vi "Waveform generation.vi"(0 "Number of Steps":dbl, 1 "488 LASER Intensity":dbl, 2 "SPIMA Obj Ampl":dbl, 3 "SPIMB Z- galvo amplitude":dbl, 4 "SPIMA Z-Galvo Offset":dbl, 5 "SPIMA Z-Galvo Amplitude":dbl, 6 "SPIMA Camera trigger":dbl, 7 "SPIMA Objective Offset":dbl, 8 "SPIMB Objective Offset":dbl, 9 "SPIMA Y-Galvo Offset":dbl, 10 "SPIMB Camera Trigger":dbl, 11 "561 Laser Amplitude":dbl, 14 "SPIMB Objective Amplitude":dbl, 15 "SPIMA Y-Galvo Amplitude":dbl, 21 "SPIMB Z-offset":dbl, 24 "SPIMB Y Offset":dbl, 25 "SPIMB Y Amplitude":dbl) -> (20 "DAQ 2":waveform(dbl)[](array[waveform]), 27 "DAQ1":waveform(dbl)[](array[waveform]))   [LabVIEW 2016]
uses:
  <vilib>/Waveform/WDTOps.llb/WDT Append Waveforms DBL.vi
  <vilib>/measure/NI_MABase.lvlib
panel:
  # "Phase 1"
  # "Phase 2"
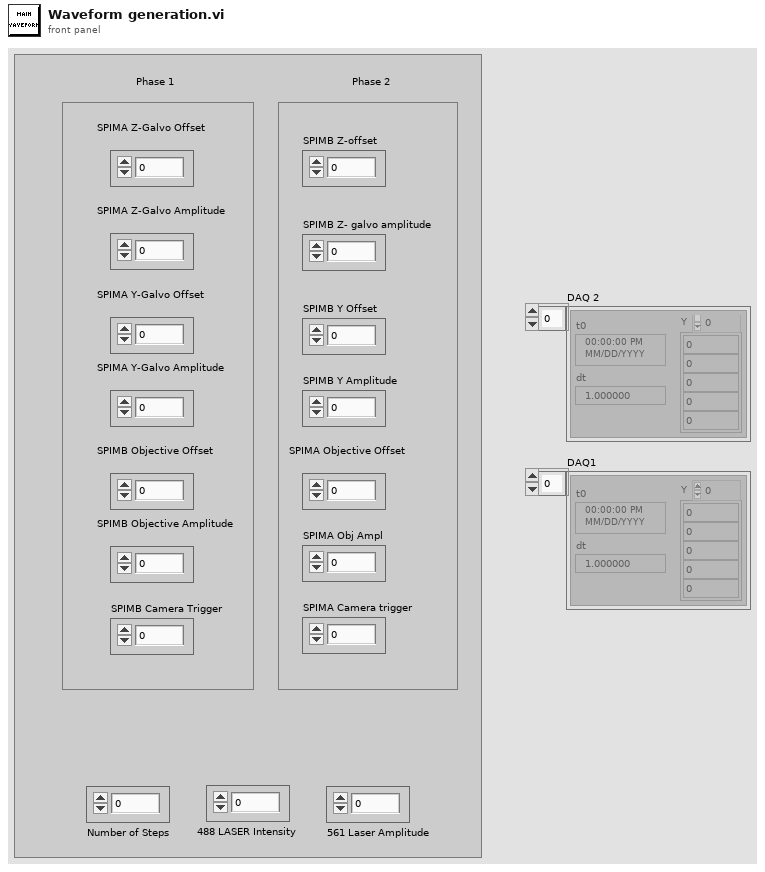
[diagram p1: front panel]
types:
  T1 = enum16{"Sine Wave", "Triangle Wave", "Square Wave", "Sawtooth Wave"}
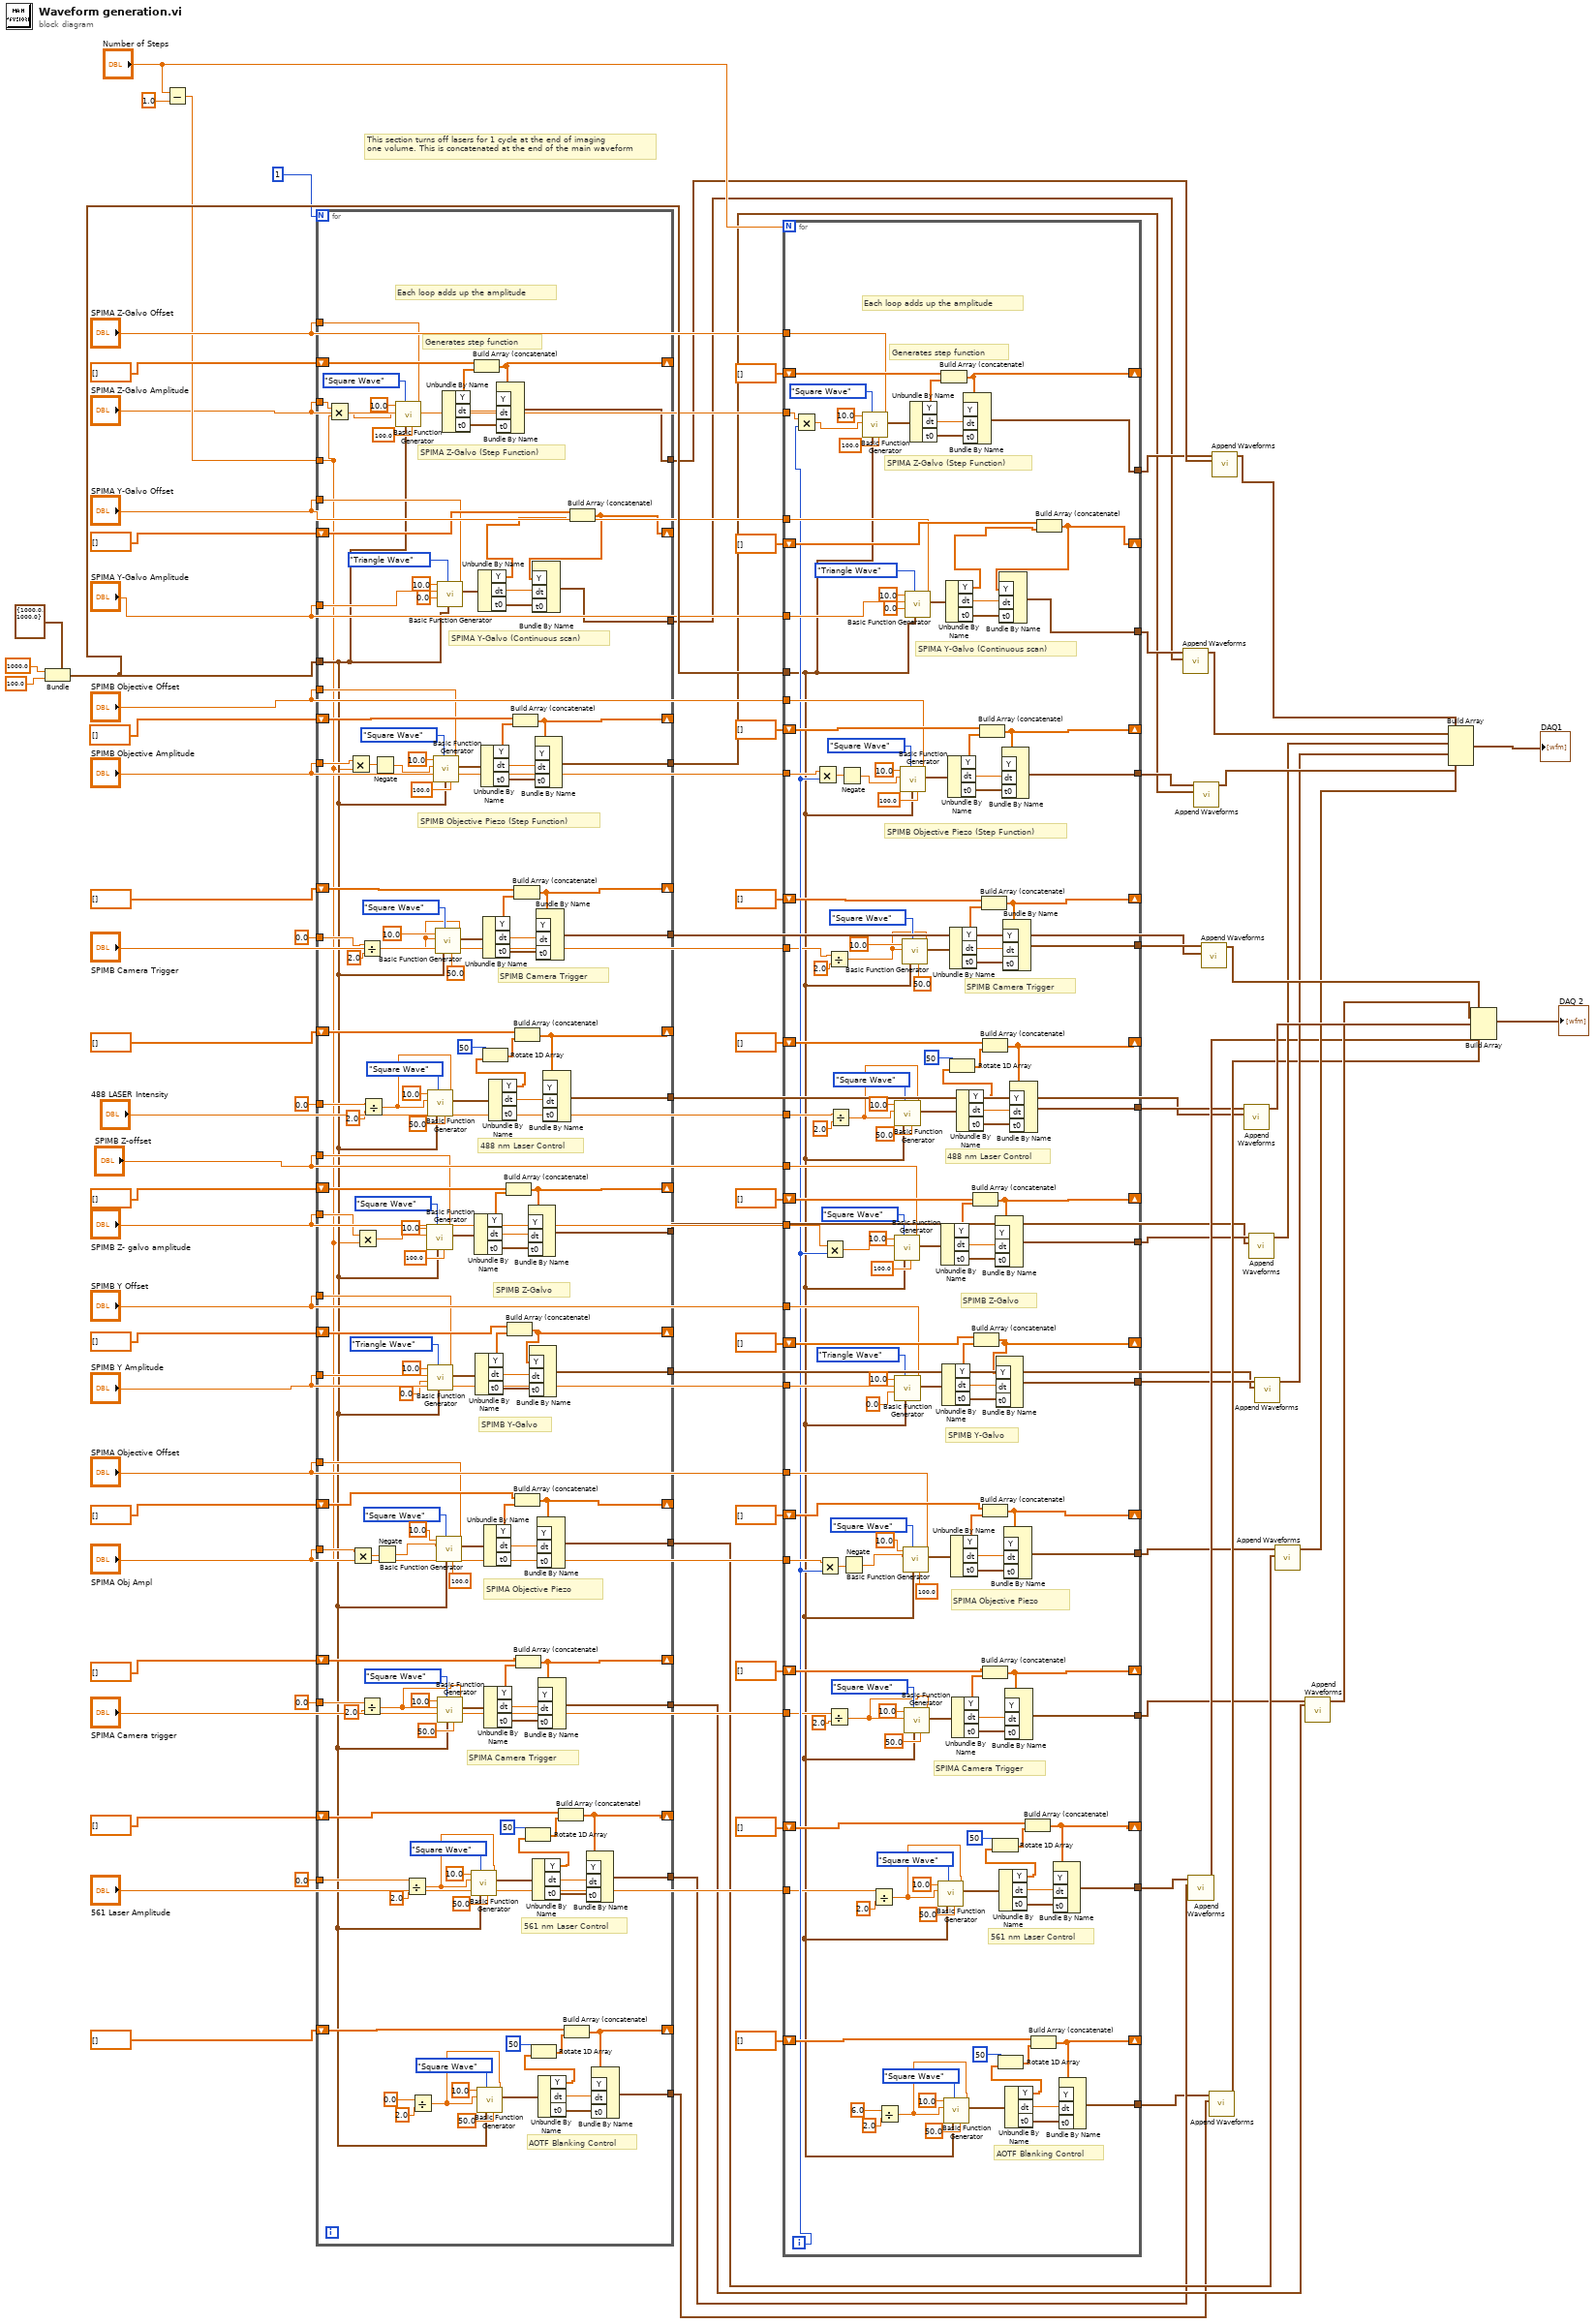
[diagram p0: block diagram]
diagram:
  # "This section turns off lasers for 1 cycle at the end of imaging\none volume. This is concatenated at the end of the main waveform"
  n1 = Bundle(cluster=cluster{"Fs":dbl, "#s":dbl} {"Fs"=1000.0, "#s"=1000.0} ("sampling info"), "Fs"=1000.0, "#s"=100.0) -> (w72:cluster{"Fs":dbl, "#s":dbl})
  n2 = Subtract(x="Number of Steps", y=1.0) -> (x-y=w29:dbl)
  n3 = for {
    N: 1 -> [_]
    shift-right: [w228] -> _
    shift-left: dbl[] [] ("appended array") -> [w229]
    tunnel: [w227] -> w22
    shift-right: [w222] -> _
    shift-left: dbl[] [] ("appended array") -> [w223]
    tunnel: [w221] -> w19
    tunnel: w72 -> [w93]
    shift-right: [w196] -> _
    shift-left: dbl[] [] ("appended array") -> [w197]
    tunnel: [w195] -> w17
    shift-right: [w193] -> _
    shift-left: dbl[] [] ("appended array") -> [w194]
    tunnel: [w192] -> w15
    tunnel: "SPIMA Z-Galvo Offset" -> [w191]
    tunnel: "SPIMA Y-Galvo Offset" -> [w190]
    tunnel: "SPIMB Objective Offset" -> [w189]
    tunnel: 0.0 ("488 LASER Intensity") -> [w141]
    tunnel: [w168] -> w11
    tunnel: [w167] -> w9
    tunnel: [w166] -> w7
    tunnel: [w165] -> w5
    shift-right: [w163] -> _
    shift-left: dbl[] [] ("appended array") -> [w164]
    shift-right: [w161] -> _
    shift-left: dbl[] [] ("appended array") -> [w162]
    shift-right: [w159] -> _
    shift-left: dbl[] [] ("appended array") -> [w160]
    shift-right: [w157] -> _
    shift-left: dbl[] [] ("appended array") -> [w158]
    tunnel: "SPIMA Z-Galvo Amplitude" -> [w156]
    tunnel: "SPIMB Objective Amplitude" -> [w154]
    tunnel: "SPIMA Y-Galvo Amplitude" -> [w152]
    tunnel: "SPIMA Objective Offset" -> [w151]
    shift-right: [w145] -> _
    shift-left: dbl[] [] ("appended array") -> [w148]
    tunnel: [w149] -> w13
    tunnel: "SPIMB Z-offset" -> [w138]
    tunnel: "SPIMB Y Offset" -> [w137]
    tunnel: "SPIMB Y Amplitude" -> [w136]
    shift-right: [w109] -> _
    shift-left: dbl[] [] ("appended array") -> [w110]
    shift-right: [w107] -> _
    shift-left: dbl[] [] ("appended array") -> [w108]
    tunnel: [w106] -> w3
    tunnel: [w105] -> w1
    tunnel: "SPIMB Z- galvo amplitude" -> [w104]
    tunnel: "SPIMA Obj Ampl" -> [w103]
    tunnel: 0.0 ("SPIMA Camera trigger") -> [w100]
    tunnel: 0.0 ("561 Laser Amplitude") -> [w97]
    tunnel: 0.0 ("SPIMB Camera Trigger") -> [w96]
    tunnel: w29 -> [w86]
    # "AOTF Blanking Control"
    # "561 nm Laser Control"
    # "Each loop adds up the amplitude"
    # "Generates step function"
    # "SPIMA Camera Trigger"
    # "SPIMA Objective Piezo"
    # "SPIMB Y-Galvo"
    # "SPIMB Z-Galvo"
    # "488 nm Laser Control"
    # "SPIMB Camera Trigger"
    # "SPIMB Objective Piezo (Step Function)"
    # "SPIMA Y-Galvo (Continuous scan)"
    # "SPIMA Z-Galvo (Step Function)"
    n4 = Multiply(x=w156, y=w86) -> (x*y=w90:dbl)
    n5 = Multiply(x=w154, y=w86) -> (x*y=w155:dbl)
    n6 = Multiply(x=w103, y=w86) -> (x*y=w102:dbl)
    n7 = Multiply(x=w104, y=w86) -> (x*y=w91:dbl)
    n8 = Divide(x=w96, y=2.0) -> (x/y=w94:dbl)
    n9 = Divide(x=w100, y=2.0) -> (x/y=w98:dbl)
    n10 = Divide(x=w141, y=2.0) -> (x/y=w139:dbl)
    n11 = Negate(x=w155) -> (-x=w153:dbl)
    n12 = Negate(x=w102) -> (-x=w101:dbl)
    n13 = call <vilib>:"Basic Function Generator.vi"("offset"=w191, "square wave duty cycle (%)"=100.0, "sampling info"=w93, "signal type"=T1."Square Wave", "amplitude"=w90, "frequency"=10.0) -> ("signal out"=w230:waveform(dbl))  [unwired: 3 in, 2 out]
    n14 = Divide(x=w97, y=2.0) -> (x/y=w125:dbl)
    n15 = Divide(x=0.0, y=2.0) -> (x/y=w114:dbl)
    n16 = call <vilib>:"Basic Function Generator.vi"("offset"=w138, "square wave duty cycle (%)"=100.0, "sampling info"=w93, "signal type"=T1."Square Wave", "amplitude"=w91, "frequency"=10.0) -> ("signal out"=w200:waveform(dbl))  [unwired: 3 in, 2 out]
    n17 = call <vilib>:"Basic Function Generator.vi"("offset"=w139, "square wave duty cycle (%)"=50.0, "sampling info"=w93, "signal type"=T1."Square Wave", "amplitude"=w139, "frequency"=10.0) -> ("signal out"=w150:waveform(dbl))  [unwired: 3 in, 2 out]
    n18 = call <vilib>:"Basic Function Generator.vi"("offset"=w137, "sampling info"=w93, "signal type"=T1."Triangle Wave", "phase"=0.0, "amplitude"=w136, "frequency"=10.0) -> ("signal out"=w185:waveform(dbl))  [unwired: 3 in, 2 out]
    n19 = call <vilib>:"Basic Function Generator.vi"("offset"=w189, "square wave duty cycle (%)"=100.0, "sampling info"=w93, "signal type"=T1."Square Wave", "amplitude"=w153, "frequency"=10.0) -> ("signal out"=w214:waveform(dbl))  [unwired: 3 in, 2 out]
    n20 = call <vilib>:"Basic Function Generator.vi"("offset"=w94, "square wave duty cycle (%)"=50.0, "sampling info"=w93, "signal type"=T1."Square Wave", "amplitude"=w94, "frequency"=10.0) -> ("signal out"=w208:waveform(dbl))  [unwired: 3 in, 2 out]
    n21 = call <vilib>:"Basic Function Generator.vi"("offset"=w151, "square wave duty cycle (%)"=100.0, "sampling info"=w93, "signal type"=T1."Square Wave", "amplitude"=w101, "frequency"=10.0) -> ("signal out"=w178:waveform(dbl))  [unwired: 3 in, 2 out]
    n22 = call <vilib>:"Basic Function Generator.vi"("offset"=w98, "square wave duty cycle (%)"=50.0, "sampling info"=w93, "signal type"=T1."Square Wave", "amplitude"=w98, "frequency"=10.0) -> ("signal out"=w171:waveform(dbl))  [unwired: 3 in, 2 out]
    n23 = call <vilib>:"Basic Function Generator.vi"("offset"=w190, "sampling info"=w93, "signal type"=T1."Triangle Wave", "phase"=0.0, "amplitude"=w152, "frequency"=10.0) -> ("signal out"=w224:waveform(dbl))  [unwired: 3 in, 2 out]
    n24 = Unbundle By Name(w230) -> ("Y"=w231:dbl[], "dt"=w219:dbl, "t0"=w220:timestamp)
    n25 = call <vilib>:"Basic Function Generator.vi"("offset"=w125, "square wave duty cycle (%)"=50.0, "sampling info"=w93, "signal type"=T1."Square Wave", "amplitude"=w125, "frequency"=10.0) -> ("signal out"=w131:waveform(dbl))  [unwired: 3 in, 2 out]
    n26 = Build Array (concatenate)(w229, w231) -> (w228:dbl[])
    n27 = Unbundle By Name(w200) -> ("Y"=w201:dbl[], "dt"=w198:dbl, "t0"=w199:timestamp)
    n28 = Unbundle By Name(w185) -> ("Y"=w186:dbl[], "dt"=w183:dbl, "t0"=w184:timestamp)
    n29 = call <vilib>:"Basic Function Generator.vi"("offset"=w114, "square wave duty cycle (%)"=50.0, "sampling info"=w93, "signal type"=T1."Square Wave", "amplitude"=w114, "frequency"=10.0) -> ("signal out"=w120:waveform(dbl))  [unwired: 3 in, 2 out]
    n30 = Unbundle By Name(w224) -> ("Y"=w87:dbl[], "dt"=w225:dbl, "t0"=w226:timestamp)
    n31 = Unbundle By Name(w214) -> ("Y"=w215:dbl[], "dt"=w212:dbl, "t0"=w213:timestamp)
    n32 = Unbundle By Name(w208) -> ("Y"=w209:dbl[], "dt"=w206:dbl, "t0"=w207:timestamp)
    n33 = Unbundle By Name(w178) -> ("Y"=w179:dbl[], "dt"=w176:dbl, "t0"=w177:timestamp)
    n34 = Unbundle By Name(w171) -> ("Y"=w172:dbl[], "dt"=w169:dbl, "t0"=w170:timestamp)
    n35 = Unbundle By Name(w150) -> ("Y"=w133:dbl[], "dt"=w147:dbl, "t0"=w146:timestamp)
    n36 = Rotate 1D Array(1:w133, 2:50 ("n")) -> (0:w134:dbl[])
    n37 = Bundle By Name("Y"=w228, "dt"=w219, "t0"=w220) -> (w227:waveform(dbl))  [unwired: 1 in]
    n38 = Build Array (concatenate)(w164, w201) -> (w163:dbl[])
    n39 = Build Array (concatenate)(w162, w186) -> (w161:dbl[])
    n40 = Build Array (concatenate)(w197, w215) -> (w196:dbl[])
    n41 = Build Array (concatenate)(w194, w209) -> (w193:dbl[])
    n42 = Build Array (concatenate)(w148, w134) -> (w145:dbl[])
    n43 = Build Array (concatenate)(w160, w179) -> (w159:dbl[])
    n44 = Build Array (concatenate)(w158, w172) -> (w157:dbl[])
    n45 = Bundle By Name("Y"=w163, "dt"=w198, "t0"=w199) -> (w168:waveform(dbl))  [unwired: 1 in]
    n46 = Bundle By Name("Y"=w161, "dt"=w183, "t0"=w184) -> (w167:waveform(dbl))  [unwired: 1 in]
    n47 = Unbundle By Name(w131) -> ("Y"=w122:dbl[], "dt"=w130:dbl, "t0"=w129:timestamp)
    n48 = Rotate 1D Array(1:w122, 2:50 ("n")) -> (0:w123:dbl[])
    n49 = Bundle By Name("Y"=w196, "dt"=w212, "t0"=w213) -> (w195:waveform(dbl))  [unwired: 1 in]
    n50 = Bundle By Name("Y"=w193, "dt"=w206, "t0"=w207) -> (w192:waveform(dbl))  [unwired: 1 in]
    n51 = Bundle By Name("Y"=w159, "dt"=w176, "t0"=w177) -> (w166:waveform(dbl))  [unwired: 1 in]
    n52 = Bundle By Name("Y"=w157, "dt"=w169, "t0"=w170) -> (w165:waveform(dbl))  [unwired: 1 in]
    n53 = Unbundle By Name(w120) -> ("Y"=w111:dbl[], "dt"=w119:dbl, "t0"=w118:timestamp)
    n54 = Rotate 1D Array(1:w111, 2:50 ("n")) -> (0:w112:dbl[])
    n55 = Bundle By Name("Y"=w145, "dt"=w147, "t0"=w146) -> (w149:waveform(dbl))  [unwired: 1 in]
    n56 = Build Array (concatenate)(w110, w123) -> (w109:dbl[])
    n57 = Build Array (concatenate)(w108, w112) -> (w107:dbl[])
    n58 = Build Array (concatenate)(w223, w87) -> (w222:dbl[])
    n59 = Bundle By Name("Y"=w222, "dt"=w225, "t0"=w226) -> (w221:waveform(dbl))  [unwired: 1 in]
    n60 = Bundle By Name("Y"=w109, "dt"=w130, "t0"=w129) -> (w106:waveform(dbl))  [unwired: 1 in]
    n61 = Bundle By Name("Y"=w107, "dt"=w119, "t0"=w118) -> (w105:waveform(dbl))  [unwired: 1 in]
  }
  n62 = for {
    N: "Number of Steps" -> [_]
    shift-right: [w379] -> _
    shift-left: dbl[] [] -> [w380]
    tunnel: [w378] -> w21
    shift-right: [w373] -> _
    shift-left: dbl[] [] -> [w374]
    tunnel: [w372] -> w20
    tunnel: w72 -> [w243]
    shift-right: [w347] -> _
    shift-left: dbl[] [] -> [w348]
    tunnel: [w346] -> w18
    shift-right: [w344] -> _
    shift-left: dbl[] [] -> [w345]
    tunnel: [w343] -> w16
    tunnel: "SPIMA Z-Galvo Offset" -> [w342]
    tunnel: "SPIMA Y-Galvo Offset" -> [w341]
    tunnel: "SPIMB Objective Offset" -> [w340]
    tunnel: "488 LASER Intensity" -> [w292]
    tunnel: [w319] -> w12
    tunnel: [w318] -> w10
    tunnel: [w317] -> w8
    tunnel: [w316] -> w6
    shift-right: [w314] -> _
    shift-left: dbl[] [] -> [w315]
    shift-right: [w312] -> _
    shift-left: dbl[] [] -> [w313]
    shift-right: [w310] -> _
    shift-left: dbl[] [] -> [w311]
    shift-right: [w308] -> _
    shift-left: dbl[] [] -> [w309]
    tunnel: "SPIMA Z-Galvo Amplitude" -> [w307]
    tunnel: "SPIMB Objective Amplitude" -> [w305]
    tunnel: "SPIMA Y-Galvo Amplitude" -> [w303]
    tunnel: "SPIMA Objective Offset" -> [w302]
    shift-right: [w296] -> _
    shift-left: dbl[] [] -> [w299]
    tunnel: [w300] -> w14
    tunnel: "SPIMB Z-offset" -> [w289]
    tunnel: "SPIMB Y Offset" -> [w288]
    tunnel: "SPIMB Y Amplitude" -> [w287]
    shift-right: [w260] -> _
    shift-left: dbl[] [] -> [w261]
    shift-right: [w258] -> _
    shift-left: dbl[] [] -> [w259]
    tunnel: [w257] -> w4
    tunnel: [w256] -> w2
    tunnel: "SPIMB Z- galvo amplitude" -> [w255]
    tunnel: "SPIMA Obj Ampl" -> [w254]
    tunnel: "SPIMA Camera trigger" -> [w250]
    tunnel: "561 Laser Amplitude" -> [w247]
    tunnel: "SPIMB Camera Trigger" -> [w246]
    i -> [w253]
    # "AOTF Blanking Control"
    # "561 nm Laser Control"
    # "Each loop adds up the amplitude"
    # "Generates step function"
    # "SPIMA Camera Trigger"
    # "SPIMA Objective Piezo"
    # "SPIMB Y-Galvo"
    # "SPIMB Z-Galvo"
    # "488 nm Laser Control"
    # "SPIMB Camera Trigger"
    # "SPIMB Objective Piezo (Step Function)"
    # "SPIMA Y-Galvo (Continuous scan)"
    # "SPIMA Z-Galvo (Step Function)"
    n63 = Multiply(x=w307, y=w253) -> (x*y=w240:dbl)
    n64 = Multiply(x=w305, y=w253) -> (x*y=w306:dbl)
    n65 = Multiply(x=w254, y=w253) -> (x*y=w252:dbl)
    n66 = Multiply(x=w255, y=w253) -> (x*y=w241:dbl)
    n67 = Divide(x=w246, y=2.0) -> (x/y=w244:dbl)
    n68 = Divide(x=w250, y=2.0) -> (x/y=w248:dbl)
    n69 = Divide(x=w292, y=2.0) -> (x/y=w290:dbl)
    n70 = Negate(x=w306) -> (-x=w304:dbl)
    n71 = Negate(x=w252) -> (-x=w251:dbl)
    n72 = call <vilib>:"Basic Function Generator.vi"("offset"=w342, "square wave duty cycle (%)"=100.0, "sampling info"=w243, "signal type"=T1."Square Wave", "amplitude"=w240, "frequency"=10.0) -> ("signal out"=w381:waveform(dbl))  [unwired: 3 in, 2 out]
    n73 = Divide(x=w247, y=2.0) -> (x/y=w276:dbl)
    n74 = Divide(x=6.0, y=2.0) -> (x/y=w265:dbl)
    n75 = call <vilib>:"Basic Function Generator.vi"("offset"=w289, "square wave duty cycle (%)"=100.0, "sampling info"=w243, "signal type"=T1."Square Wave", "amplitude"=w241, "frequency"=10.0) -> ("signal out"=w351:waveform(dbl))  [unwired: 3 in, 2 out]
    n76 = call <vilib>:"Basic Function Generator.vi"("offset"=w290, "square wave duty cycle (%)"=50.0, "sampling info"=w243, "signal type"=T1."Square Wave", "amplitude"=w290, "frequency"=10.0) -> ("signal out"=w301:waveform(dbl))  [unwired: 3 in, 2 out]
    n77 = call <vilib>:"Basic Function Generator.vi"("offset"=w288, "sampling info"=w243, "signal type"=T1."Triangle Wave", "phase"=0.0, "amplitude"=w287, "frequency"=10.0) -> ("signal out"=w336:waveform(dbl))  [unwired: 3 in, 2 out]
    n78 = call <vilib>:"Basic Function Generator.vi"("offset"=w340, "square wave duty cycle (%)"=100.0, "sampling info"=w243, "signal type"=T1."Square Wave", "amplitude"=w304, "frequency"=10.0) -> ("signal out"=w365:waveform(dbl))  [unwired: 3 in, 2 out]
    n79 = call <vilib>:"Basic Function Generator.vi"("offset"=w244, "square wave duty cycle (%)"=50.0, "sampling info"=w243, "signal type"=T1."Square Wave", "amplitude"=w244, "frequency"=10.0) -> ("signal out"=w359:waveform(dbl))  [unwired: 3 in, 2 out]
    n80 = call <vilib>:"Basic Function Generator.vi"("offset"=w302, "square wave duty cycle (%)"=100.0, "sampling info"=w243, "signal type"=T1."Square Wave", "amplitude"=w251, "frequency"=10.0) -> ("signal out"=w329:waveform(dbl))  [unwired: 3 in, 2 out]
    n81 = call <vilib>:"Basic Function Generator.vi"("offset"=w248, "square wave duty cycle (%)"=50.0, "sampling info"=w243, "signal type"=T1."Square Wave", "amplitude"=w248, "frequency"=10.0) -> ("signal out"=w322:waveform(dbl))  [unwired: 3 in, 2 out]
    n82 = call <vilib>:"Basic Function Generator.vi"("offset"=w341, "sampling info"=w243, "signal type"=T1."Triangle Wave", "phase"=0.0, "amplitude"=w303, "frequency"=10.0) -> ("signal out"=w375:waveform(dbl))  [unwired: 3 in, 2 out]
    n83 = Unbundle By Name(w381) -> ("Y"=w382:dbl[], "dt"=w370:dbl, "t0"=w371:timestamp)
    n84 = call <vilib>:"Basic Function Generator.vi"("offset"=w276, "square wave duty cycle (%)"=50.0, "sampling info"=w243, "signal type"=T1."Square Wave", "amplitude"=w276, "frequency"=10.0) -> ("signal out"=w282:waveform(dbl))  [unwired: 3 in, 2 out]
    n85 = Build Array (concatenate)(w380, w382) -> (w379:dbl[])
    n86 = Unbundle By Name(w351) -> ("Y"=w352:dbl[], "dt"=w349:dbl, "t0"=w350:timestamp)
    n87 = Unbundle By Name(w336) -> ("Y"=w337:dbl[], "dt"=w334:dbl, "t0"=w335:timestamp)
    n88 = call <vilib>:"Basic Function Generator.vi"("offset"=w265, "square wave duty cycle (%)"=50.0, "sampling info"=w243, "signal type"=T1."Square Wave", "amplitude"=w265, "frequency"=10.0) -> ("signal out"=w271:waveform(dbl))  [unwired: 3 in, 2 out]
    n89 = Unbundle By Name(w375) -> ("Y"=w237:dbl[], "dt"=w376:dbl, "t0"=w377:timestamp)
    n90 = Unbundle By Name(w365) -> ("Y"=w366:dbl[], "dt"=w363:dbl, "t0"=w364:timestamp)
    n91 = Unbundle By Name(w359) -> ("Y"=w360:dbl[], "dt"=w357:dbl, "t0"=w358:timestamp)
    n92 = Unbundle By Name(w329) -> ("Y"=w330:dbl[], "dt"=w327:dbl, "t0"=w328:timestamp)
    n93 = Unbundle By Name(w322) -> ("Y"=w323:dbl[], "dt"=w320:dbl, "t0"=w321:timestamp)
    n94 = Unbundle By Name(w301) -> ("Y"=w284:dbl[], "dt"=w298:dbl, "t0"=w297:timestamp)
    n95 = Rotate 1D Array(1:w284, 2:50 ("n")) -> (0:w285:dbl[])
    n96 = Bundle By Name("Y"=w379, "dt"=w370, "t0"=w371) -> (w378:waveform(dbl))  [unwired: 1 in]
    n97 = Build Array (concatenate)(w315, w352) -> (w314:dbl[])
    n98 = Build Array (concatenate)(w313, w337) -> (w312:dbl[])
    n99 = Build Array (concatenate)(w348, w366) -> (w347:dbl[])
    n100 = Build Array (concatenate)(w345, w360) -> (w344:dbl[])
    n101 = Build Array (concatenate)(w299, w285) -> (w296:dbl[])
    n102 = Build Array (concatenate)(w311, w330) -> (w310:dbl[])
    n103 = Build Array (concatenate)(w309, w323) -> (w308:dbl[])
    n104 = Bundle By Name("Y"=w314, "dt"=w349, "t0"=w350) -> (w319:waveform(dbl))  [unwired: 1 in]
    n105 = Bundle By Name("Y"=w312, "dt"=w334, "t0"=w335) -> (w318:waveform(dbl))  [unwired: 1 in]
    n106 = Unbundle By Name(w282) -> ("Y"=w273:dbl[], "dt"=w281:dbl, "t0"=w280:timestamp)
    n107 = Rotate 1D Array(1:w273, 2:50 ("n")) -> (0:w274:dbl[])
    n108 = Bundle By Name("Y"=w347, "dt"=w363, "t0"=w364) -> (w346:waveform(dbl))  [unwired: 1 in]
    n109 = Bundle By Name("Y"=w344, "dt"=w357, "t0"=w358) -> (w343:waveform(dbl))  [unwired: 1 in]
    n110 = Bundle By Name("Y"=w310, "dt"=w327, "t0"=w328) -> (w317:waveform(dbl))  [unwired: 1 in]
    n111 = Bundle By Name("Y"=w308, "dt"=w320, "t0"=w321) -> (w316:waveform(dbl))  [unwired: 1 in]
    n112 = Unbundle By Name(w271) -> ("Y"=w262:dbl[], "dt"=w270:dbl, "t0"=w269:timestamp)
    n113 = Rotate 1D Array(1:w262, 2:50 ("n")) -> (0:w263:dbl[])
    n114 = Bundle By Name("Y"=w296, "dt"=w298, "t0"=w297) -> (w300:waveform(dbl))  [unwired: 1 in]
    n115 = Build Array (concatenate)(w261, w274) -> (w260:dbl[])
    n116 = Build Array (concatenate)(w259, w263) -> (w258:dbl[])
    n117 = Build Array (concatenate)(w374, w237) -> (w373:dbl[])
    n118 = Bundle By Name("Y"=w373, "dt"=w376, "t0"=w377) -> (w372:waveform(dbl))  [unwired: 1 in]
    n119 = Bundle By Name("Y"=w260, "dt"=w281, "t0"=w280) -> (w257:waveform(dbl))  [unwired: 1 in]
    n120 = Bundle By Name("Y"=w258, "dt"=w270, "t0"=w269) -> (w256:waveform(dbl))  [unwired: 1 in]
  }
  n121 = call-poly <vilib>:"Append Waveforms.vi"("waveform B"=w19, "waveform A"=w20) -> ("waveform out"=w45:waveform(dbl))  [unwired: 8 in, 1 out]
  n122 = call-poly <vilib>:"Append Waveforms.vi"("waveform B"=w3, "waveform A"=w4) -> ("waveform out"=w37:waveform(dbl))  [unwired: 8 in, 1 out]
  n123 = call-poly <vilib>:"Append Waveforms.vi"("waveform B"=w17, "waveform A"=w18) -> ("waveform out"=w44:waveform(dbl))  [unwired: 8 in, 1 out]
  n124 = call-poly <vilib>:"Append Waveforms.vi"("waveform B"=w15, "waveform A"=w16) -> ("waveform out"=w43:waveform(dbl))  [unwired: 8 in, 1 out]
  n125 = call-poly <vilib>:"Append Waveforms.vi"("waveform B"=w1, "waveform A"=w2) -> ("waveform out"=w36:waveform(dbl))  [unwired: 8 in, 1 out]
  n126 = call-poly <vilib>:"Append Waveforms.vi"("waveform B"=w22, "waveform A"=w21) -> ("waveform out"=w46:waveform(dbl))  [unwired: 8 in, 1 out]
  n127 = call-poly <vilib>:"Append Waveforms.vi"("waveform B"=w13, "waveform A"=w14) -> ("waveform out"=w42:waveform(dbl))  [unwired: 8 in, 1 out]
  n128 = call-poly <vilib>:"Append Waveforms.vi"("waveform B"=w11, "waveform A"=w12) -> ("waveform out"=w41:waveform(dbl))  [unwired: 8 in, 1 out]
  n129 = call-poly <vilib>:"Append Waveforms.vi"("waveform B"=w9, "waveform A"=w10) -> ("waveform out"=w40:waveform(dbl))  [unwired: 8 in, 1 out]
  n130 = call-poly <vilib>:"Append Waveforms.vi"("waveform B"=w7, "waveform A"=w8) -> ("waveform out"=w39:waveform(dbl))  [unwired: 8 in, 1 out]
  n131 = call-poly <vilib>:"Append Waveforms.vi"("waveform B"=w5, "waveform A"=w6) -> ("waveform out"=w38:waveform(dbl))  [unwired: 8 in, 1 out]
  n132 = Build Array(w46, w45, w41, w40, w44, w39) -> (→"DAQ1":waveform(dbl)[])
  n133 = Build Array(w43, w38, w42, w37, w36) -> (→"DAQ 2":waveform(dbl)[])
